vi "xmlEdit.vi"(0 "xml路径":path, 1 "错误输入":errorcluster, 2 "tagID":string="Outcome", 3 "tagID index":i32, 5 "attibutes index":i32, 6 "new value":string) -> (4 "错误输出":errorcluster, 7 "loaded":bool, 8 "saved?":bool)   [LabVIEW 2011]
panel:
  in  "MSXML2.IXMLDOMDocument2":refnum<k7>
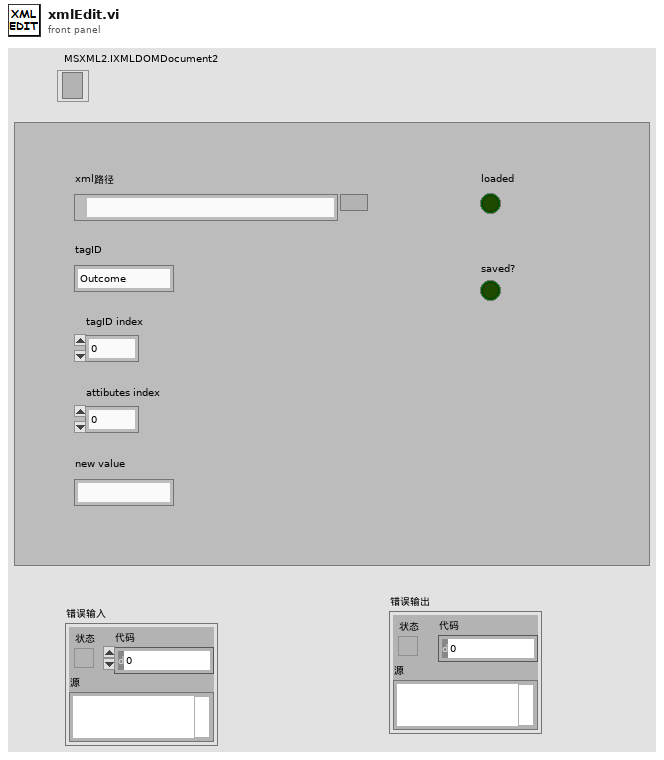
[diagram p1: front panel]
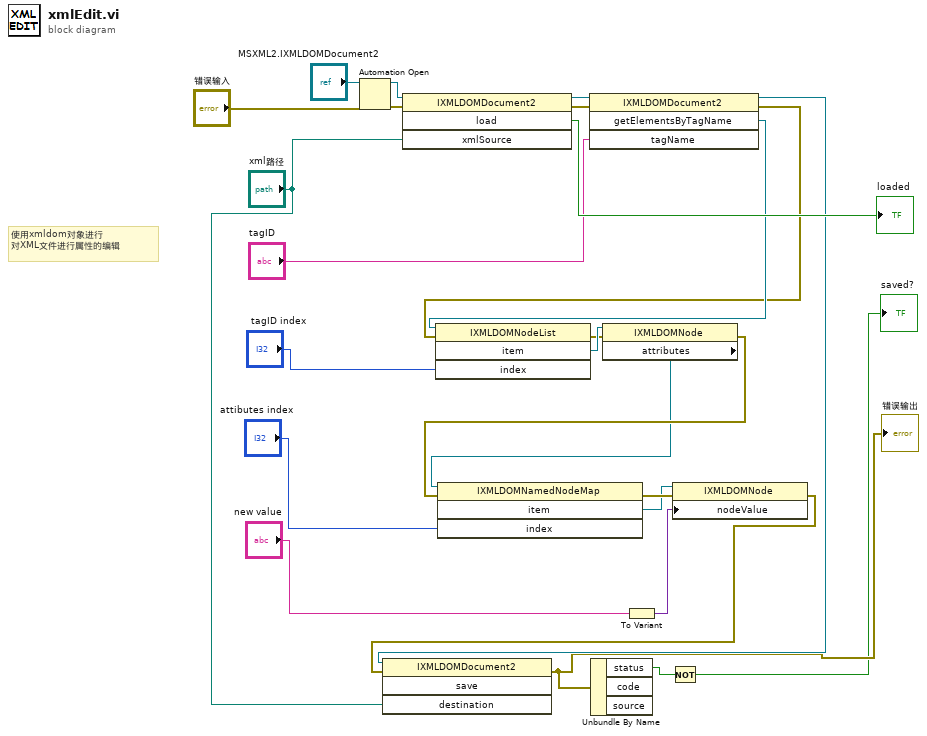
[diagram p0: block diagram]
diagram:
  # "使用xmldom对象进行\n对XML文件进行属性的编辑"
  n1 = Automation Open(error in (no error)="错误输入", Automation Refnum="MSXML2.IXMLDOMDocument2") -> (Automation Refnum=w25:refnum<k7>, error out=w15:errorcluster)  [unwired: 2 in]
  n2 = invoke class="IXMLDOMDocument2" method="load"(reference=w25, error in=w15, "xmlSource"="xml路径") -> (reference out=w23:refnum<k7>, error out=w14:errorcluster, "load"=→"loaded":bool)  [unwired: 1 in, 1 out]
  n3 = invoke class="IXMLDOMDocument2" method="getElementsByTagName"(reference=w23, error in=w14, "tagName"="tagID") -> (reference out=w10:refnum<k7>, error out=w13:errorcluster, "getElementsByTagName"=w22:refnum<k7>)  [unwired: 1 in, 1 out]
  n4 = invoke class="IXMLDOMNodeList" method="item"(reference=w22, error in=w13, "index"="tagID index") -> (error out=w12:errorcluster, "item"=w20:refnum<k7>)  [unwired: 1 in, 2 out]
  n5 = property class="IXMLDOMNode"(reference=w20, error in=w12) -> (error out=w11:errorcluster, "attributes"=w3:refnum<k7>)  [unwired: 1 out]
  n6 = invoke class="IXMLDOMNamedNodeMap" method="item"(reference=w3, error in=w11, "index"="attibutes index") -> (error out=w19:errorcluster, "item"=w18:refnum<k7>)  [unwired: 1 in, 2 out]
  n7 = To Variant(anything="new value") -> (Variant=w16:variant)
  n8 = property class="IXMLDOMNode"(reference=w18, error in=w19, "nodeValue"=w16) -> (error out=w9:errorcluster)  [unwired: 1 out]
  n9 = invoke class="IXMLDOMDocument2" method="save"(reference=w10, error in=w9, "destination"="xml路径") -> (error out=w6:errorcluster)  [unwired: 1 in, 3 out]
  "错误输出" <- w6
  n10 = Unbundle By Name(w6) -> ("status"=w5:bool)  [unwired: 2 out]
  n11 = Not(x=w5) -> (.not. x?=→"saved?":bool)
